vi "Cache Config.vi"(8 "error in (no error)":errorcluster, 11 "Security in":refnum<class "Security.lvclass">) -> (0 "error out":errorcluster, 3 "Security out":refnum<class "Security.lvclass">)   [LabVIEW 2020, in "HTTP Server.lvlib" / "Security.lvclass"]
uses:
  Security.lvclass
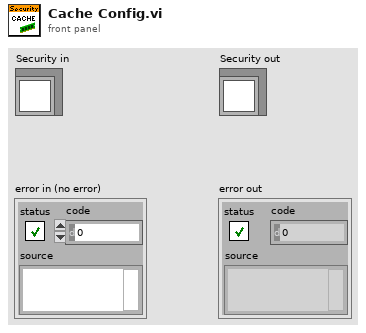
[diagram p1: front panel]
types:
  T1 = typedef "HTTP Server.lvlib/Security.lvclass/Ref Data.ctl" = cluster{"Hierarchy":T2}
  T2 = typedef "HTTP Server.lvlib/Security.lvclass/Hierarchy.ctl" = map{string, set{string}}
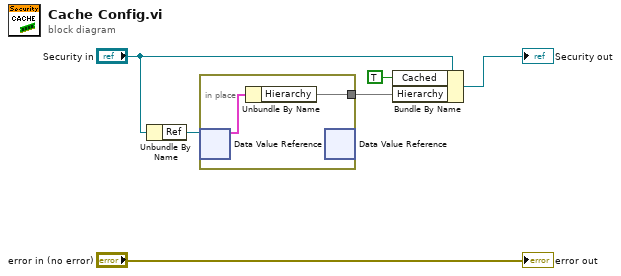
[diagram p0: block diagram]
diagram:
  n1 = Unbundle By Name("Security in") -> ("Ref"=w5:refnum<data-value>)
  n2 = in-place {
    in-place-border: [w7] -> w4
    n3 = in-place-dvr #1(w5) -> (w8:T1)  [unwired: 1 out]
    n4 = Unbundle By Name(w8) -> ("Hierarchy"=w7:T2)
    n5 = in-place-dvr #1() -> ()  [unwired: 1 in, 2 out]
  }
  n6 = Bundle By Name(cluster="Security in", "Cached"=TRUE, "Hierarchy"=w4) -> (→"Security out":refnum<class "Security.lvclass">)
  "error out" <- "error in (no error)"
